vi "VISA read.vi"(8 "error in (no error)":errorcluster, 11 "AOTF in":refnum<class "Invivo_AOTF.lvclass">) -> (0 "error out":errorcluster, 2 "buffer out":string, 3 "AOTF out":refnum<class "Invivo_AOTF.lvclass">)   [LabVIEW 2012, in "Invivo_AOTF.lvclass"]
uses:
  Invivo_AOTF.lvclass
  Invivo_AOTF.lvclass/Invivo_AOTF.ctl
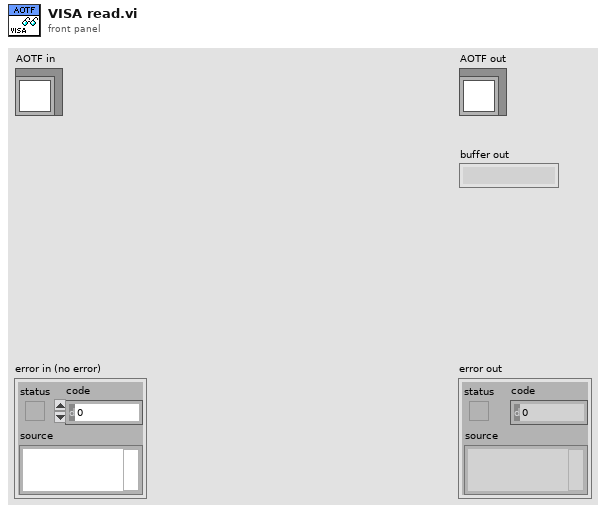
[diagram p1: front panel]
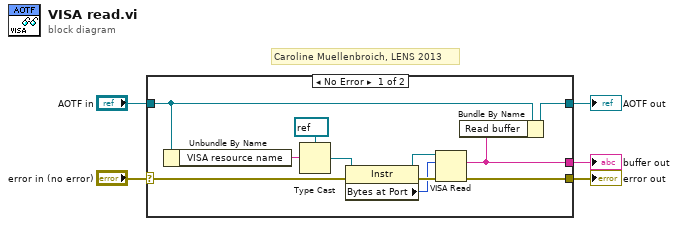
[diagram p0: block diagram]
diagram:
  # "Caroline Muellenbroich, LENS 2013"
  n1 = case shown="No Error" "error in (no error)" {
    selector: "error in (no error)" -> [w13 w18]
    tunnel: [w12 w18] -> w4
    tunnel: [w7 w17] -> w2
    tunnel: "AOTF in" -> [w8 w17]
    tunnel: [w6 _] -> w1
    frame No Error {
      n2 = Unbundle By Name(w8) -> ("VISA resource name"=w10:string)
      n3 = Type Cast(type=refnum<visa-resource-name> refnum ("reference"), x=w10) -> (*(type *) &x=w9:refnum<visa-resource-name>)
      n4 = property class="Instr"(reference=w9, error in=w13) -> (reference out=w15:refnum<visa-resource-name>, error out=w16:errorcluster, "Bytes at Port"=w14:u32)
      n5 = VISA Read(VISA resource name=w15, byte count=w14, error in (no error)=w16) -> (read buffer=w6:string, error out=w12:errorcluster)  [unwired: 2 out]
      n6 = Bundle By Name(cluster=w8, "Read buffer"=w6) -> (w7:refnum<class "Invivo_AOTF.lvclass">)
    }
    frame Error {
    }
  }
  "error out" <- w4
  "AOTF out" <- w2
  "buffer out" <- w1
